vi "Read_PICO.vi"() -> ()   [LabVIEW 2024]
uses:
  <vilib>/Instr/_visa.llb/VISA Configure Serial Port (Instr).vi
panel:
  out "Tecla Ingresada":string
  out "duty":i32
  out "Acc":i32
  out "Temperatura":dbl
  out "lamp":i32
  out "ir_string":i32
  out "dark":i32
  out "bulb":i32
  out "Estado de Acceso":string
  out "Gauge":dbl(knob) scale=0.0..100.0
  out "Thermometer":dbl(slide) scale=0.0..100.0
  out "IR":bool
  out "LDR":bool
  out "?":dbl(graph)
  out "LED 3 Claps":bool
  out "LED 2 Claps":bool
  in  "stop":bool
  in  "Baud Rate (115200)":dbl
  in  "VISA resource name":refnum<visa-resource-name>
  out "Read buffer":string
  # "Proyecto DomoSync. Casa Domótica. \nAcondicionamiento de Señales - Electrónica Digital III"
  # "Luz habitación"
  # "Luz Lámpara"
  # "Ambiente Oscuro"
  # "Infrarrojo"
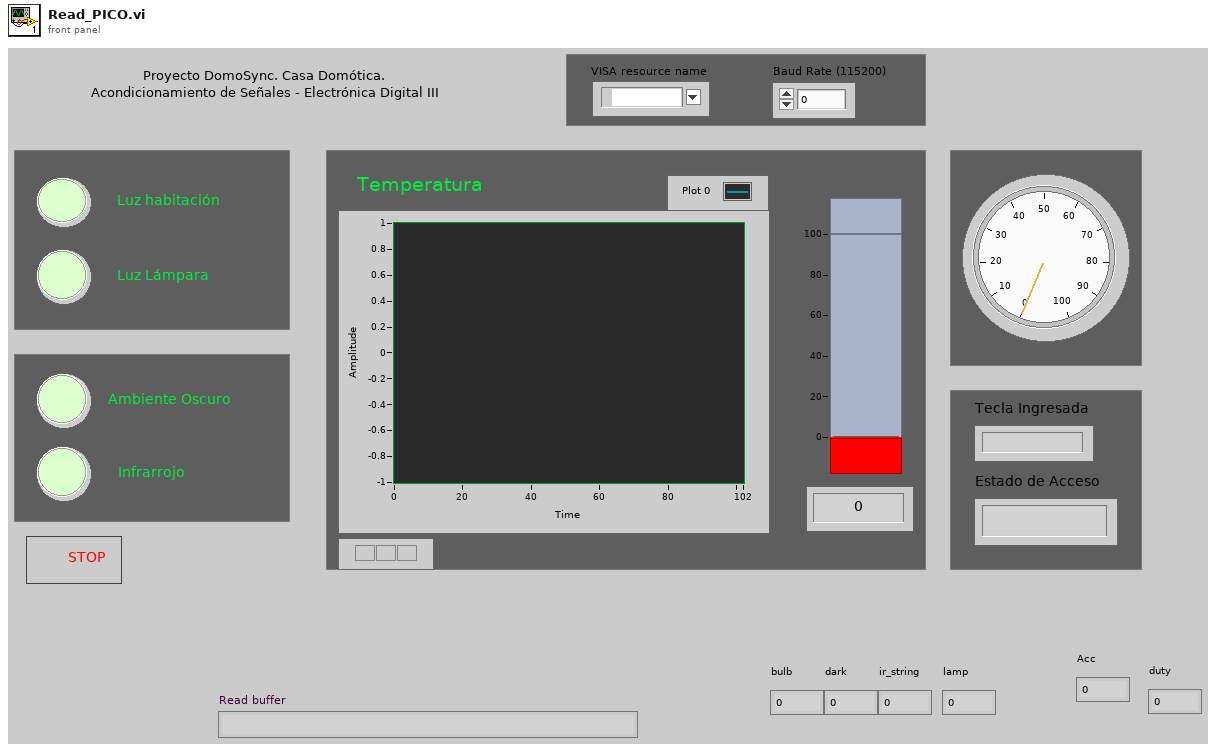
[diagram p1: front panel]
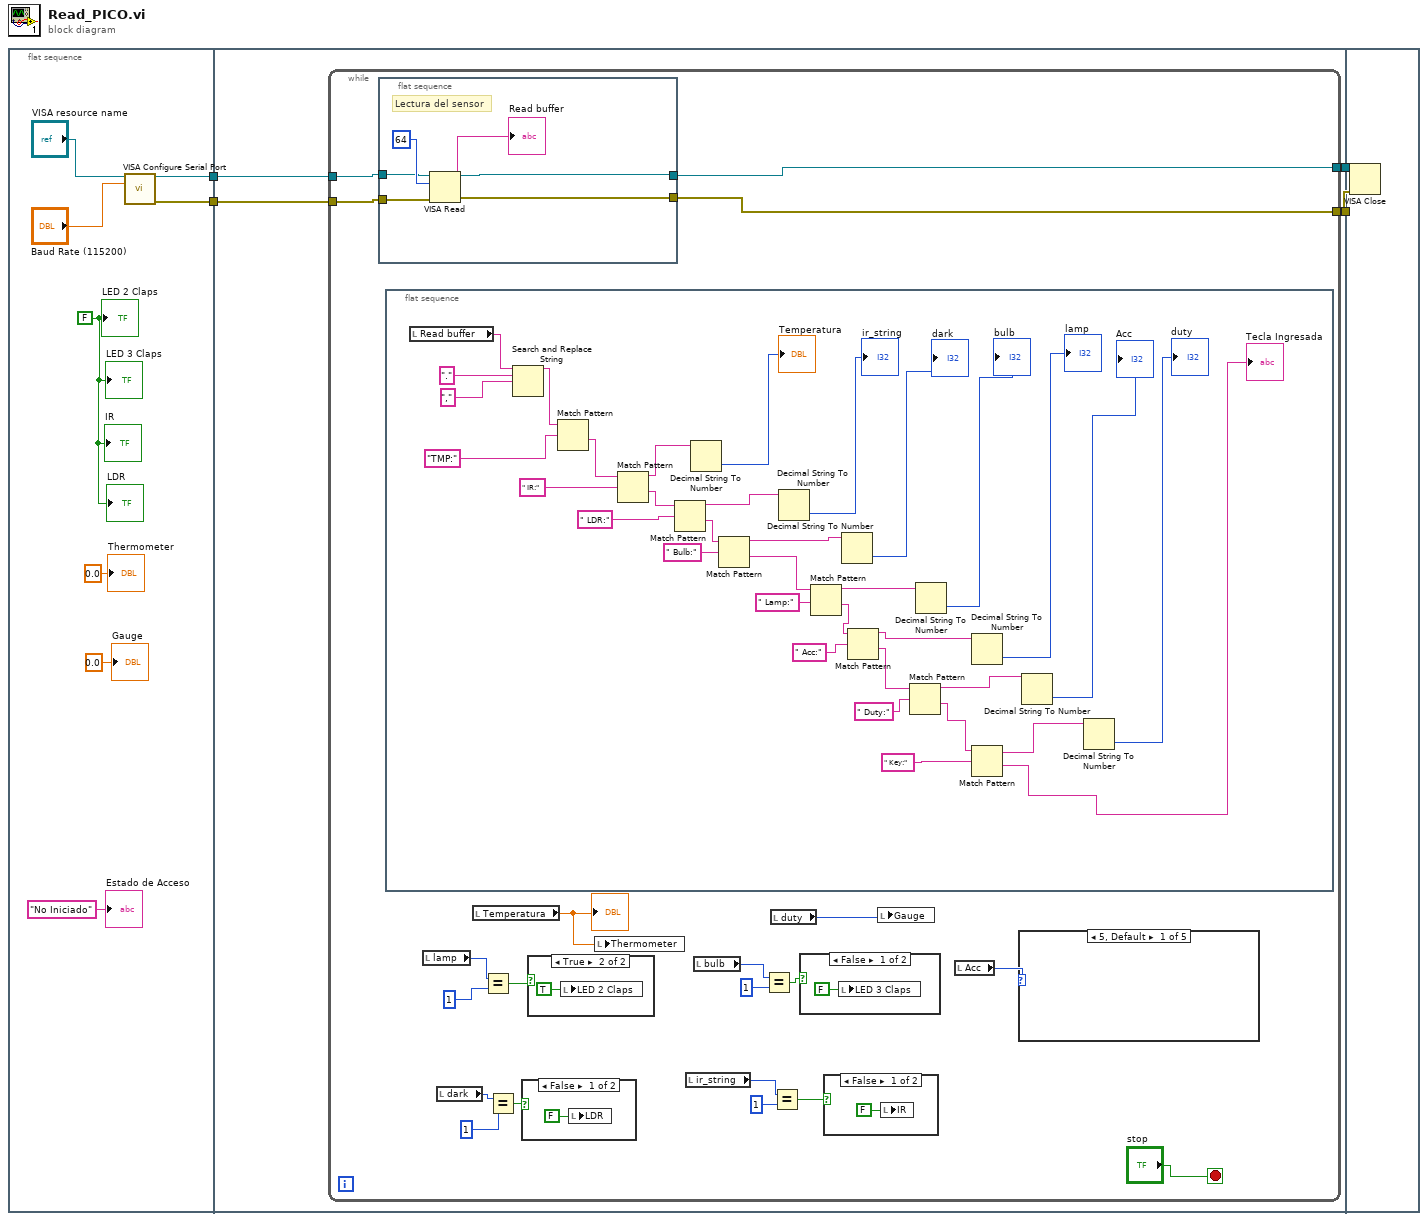
[diagram p0: block diagram]
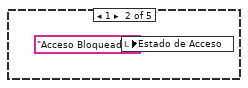
[diagram p2: hidden frame]
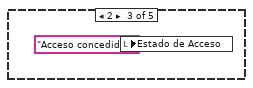
[diagram p3: hidden frame]
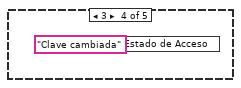
[diagram p4: hidden frame]
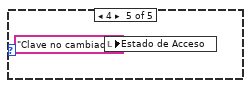
[diagram p5: hidden frame]
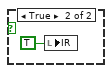
[diagram p6: hidden frame]
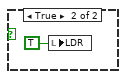
[diagram p7: hidden frame]
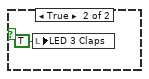
[diagram p8: hidden frame]
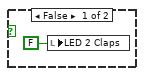
[diagram p9: hidden frame]
diagram:
  n1 = flat-sequence {
    tunnel: [w10] -> w4
    tunnel: [w9] -> w1
    tunnel: w4 -> [w16]
    tunnel: [w15] -> w3
    tunnel: [w14] -> w2
    tunnel: w1 -> [w13]
    tunnel: w3 -> [w90]
    tunnel: w2 -> [w89]
    frame #0 {
      w8 = FALSE ("LED 2 Claps")
      n2 = call-poly "VISA Configure Serial Port"("VISA resource name"="VISA resource name", "baud rate (9600)"="Baud Rate (115200)") -> ("VISA resource name out"=w10:refnum<visa-resource-name>, "error out"=w9:errorcluster)  [unwired: 12 in]
      "IR" <- w8
      "LDR" <- w8
      "LED 2 Claps" <- w8
      "LED 3 Claps" <- w8
      "Thermometer" <- 0.0 ("Thermometer")
      "Gauge" <- 0.0 ("Gauge")
      "Estado de Acceso" <- "No Iniciado" ("Access")
    }
    frame #1 {
      n3 = while {
        tunnel: w16 -> [w36]
        tunnel: [w35] -> w15
        tunnel: [w34] -> w14
        tunnel: w13 -> [w33]
        stop <- "stop" stop-if-true
        n4 = flat-sequence {
          tunnel: w36 -> [w87]
          tunnel: w33 -> [w86]
          tunnel: [w85] -> w35
          tunnel: [w84] -> w34
          frame #0 {
            # "Lectura del sensor"
            n5 = VISA Read(VISA resource name=w87, byte count=64, error in (no error)=w86) -> (VISA resource name out=w85:refnum<visa-resource-name>, read buffer=→"Read buffer":string, error out=w84:errorcluster)  [unwired: 1 out]
          }
        }
        n6 = flat-sequence {
          frame #0 {
            n7 = local read "Read buffer"() -> (w82:string)
            n8 = Search and Replace String(input string=w82, search string=".", replace string="," ("replace string (\"\")")) -> (result string=w81:string)  [unwired: 5 in, 3 out]
            n9 = Match Pattern(string=w81, regular expression="TMP:") -> (after substring=w76:string)  [unwired: 1 in, 3 out]
            n10 = Match Pattern(string=w76, regular expression=" IR:") -> (before substring=w73:string, after substring=w77:string)  [unwired: 1 in, 2 out]
            n11 = Match Pattern(string=w77, regular expression=" LDR:") -> (before substring=w72:string, after substring=w75:string)  [unwired: 1 in, 2 out]
            n12 = Decimal String To Number(string=w73) -> (number=→"Temperatura":i32)  [unwired: 2 in, 1 out]
            n13 = Match Pattern(string=w75, regular expression=" Bulb:") -> (before substring=w71:string, after substring=w66:string)  [unwired: 1 in, 2 out]
            n14 = Decimal String To Number(string=w72) -> (number=→"ir_string":i32)  [unwired: 2 in, 1 out]
            n15 = Match Pattern(string=w66, regular expression=" Lamp:") -> (before substring=w70:string, after substring=w63:string)  [unwired: 1 in, 2 out]
            n16 = Decimal String To Number(string=w71) -> (number=→"dark":i32)  [unwired: 2 in, 1 out]
            n17 = Match Pattern(string=w63, regular expression=" Acc:") -> (before substring=w61:string, after substring=w62:string)  [unwired: 1 in, 2 out]
            n18 = Match Pattern(string=w62, regular expression=" Duty:") -> (before substring=w54:string, after substring=w52:string)  [unwired: 1 in, 2 out]
            n19 = Decimal String To Number(string=w70) -> (number=→"bulb":i32)  [unwired: 2 in, 1 out]
            n20 = Decimal String To Number(string=w61) -> (number=→"lamp":i32)  [unwired: 2 in, 1 out]
            n21 = Match Pattern(string=w52, regular expression=" Key:") -> (before substring=w51:string, after substring=→"Tecla Ingresada":string)  [unwired: 1 in, 2 out]
            n22 = Decimal String To Number(string=w54) -> (number=→"Acc":i32)  [unwired: 2 in, 1 out]
            n23 = Decimal String To Number(string=w51) -> (number=→"duty":i32)  [unwired: 2 in, 1 out]
          }
        }
        n24 = local read "lamp"() -> (w23:i32)
        n25 = local read "dark"() -> (w24:i32)
        n26 = local read "Temperatura"() -> (w22:dbl)
        "?" <- w22
        n27 = Equal?(x=w23, y=1) -> (x = y?=w31:bool)
        n28 = Equal?(x=w24, y=1) -> (x = y?=w19:bool)
        n29 = case shown="False" w19 {
          frame False {
            n30 = local write "LDR"(FALSE ("LDR")) -> ()
          }
          frame True {
            n31 = local write "LDR"(TRUE ("LDR")) -> ()
          }
        }
        n32 = case shown="True" w31 {
          frame False {
            n33 = local write "LED 2 Claps"(FALSE ("LED 2 Claps")) -> ()
          }
          frame True {
            n34 = local write "LED 2 Claps"(TRUE ("LED 2 Claps")) -> ()
          }
        }
        n35 = local write "Thermometer"(w22) -> ()
        n36 = local read "ir_string"() -> (w25:i32)
        n37 = local read "bulb"() -> (w26:i32)
        n38 = Equal?(x=w26, y=1) -> (x = y?=w21:bool)
        n39 = local read "duty"() -> (w17:i32)
        n40 = Equal?(x=w25, y=1) -> (x = y?=w20:bool)
        n41 = case shown="False" w21 {
          frame False {
            n42 = local write "LED 3 Claps"(FALSE ("LED 3 Claps")) -> ()
          }
          frame True {
            n43 = local write "LED 3 Claps"(TRUE ("LED 3 Claps")) -> ()
          }
        }
        n44 = case shown="False" w20 {
          frame False {
            n45 = local write "IR"(FALSE ("IR")) -> ()
          }
          frame True {
            n46 = local write "IR"(TRUE ("IR")) -> ()
          }
        }
        n47 = local write "Gauge"(w17) -> ()
        n48 = local read "Acc"() -> (w18:i32)
        n49 = case shown="5, Default" w18 {
          frame 5, Default {
          }
          frame 1 {
            n50 = local write "Estado de Acceso"("Acceso Bloqueado" ("Access")) -> ()
          }
          frame 2 {
            n51 = local write "Estado de Acceso"("Acceso concedido" ("Access")) -> ()
          }
          frame 3 {
            n52 = local write "Estado de Acceso"("Clave cambiada" ("Access")) -> ()
          }
          frame 4 {
            n53 = local write "Estado de Acceso"("Clave no cambiada" ("Access")) -> ()
          }
        }
      }
    }
    frame #2 {
      n54 = VISA Close(VISA resource name=w90, error in (no error)=w89) -> ()  [unwired: 1 out]
    }
  }
